vi "instantiate_text_files_source.vi"(0 "text files":path[](array[path]), 11 "error in (no error)":errorcluster) -> (4 "datasource_text_file out":refnum<class "datasource_text_file.lvclass">, 15 "error out":errorcluster)   [LabVIEW 2020, in "datasource_text_file.lvclass"]
uses:
  datasource_text_file.lvclass
  datasource_text_file.lvclass/datasource_text_file.ctl
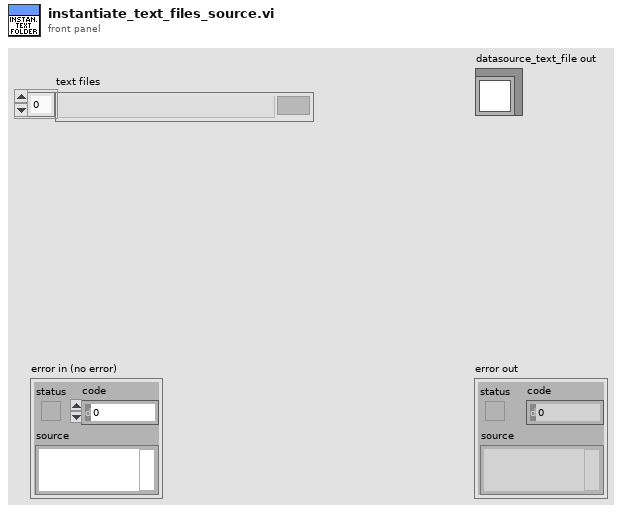
[diagram p1: front panel]
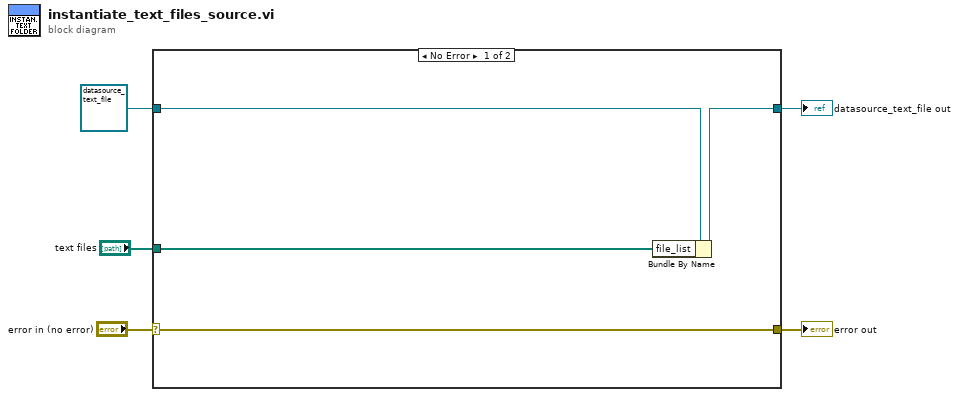
[diagram p0: block diagram]
diagram:
  n1 = case shown="No Error" "error in (no error)" {
    selector: "error in (no error)" -> [w7 w11]
    tunnel: [w7 w11] -> w4
    tunnel: [w8 w10] -> w2
    tunnel: refnum<class "datasource_text_file.lvclass"> refnum ("datasource_text_file in") -> [w9 w10]
    tunnel: "text files" -> [w6 _]
    frame No Error {
      n2 = Bundle By Name(cluster=w9, "file_list"=w6) -> (w8:refnum<class "datasource_text_file.lvclass">)
    }
    frame Error {
    }
  }
  "error out" <- w4
  "datasource_text_file out" <- w2
